vi "com_test.vi"() -> ()   [LabVIEW 2012]
uses:
  <vilib>/Analysis/2dsp.llb/1D Auto Correlation (CDB).vi
  <vilib>/Analysis/2dsp.llb/1D Cross Correlation (CDB).vi
  <vilib>/Analysis/NI_AALPro.lvlib
panel:
  out "Transmitted signal":dbl[](graph)
  out "Transmitted symbols autocorrelation":dbl[](graph)
  out "Transmitted and received symbols Xcorrelation":dbl[](graph)
  out "error out":errorcluster
  in  "RX Parameters":T1={"RX Oversample Factor"=4, "RX Sample Rate"=4000000.0, "Synchronization Options"={"Synchronization Method"=enum."Timing Estimation", "Symbol Timing Recovery Method "=enum."Maximum Energy", "Fixed Offset"=0.0, "Frame Detection Method"=enum."", "Correct Frequency Offset"=FALSE}, "Channel Estimation/Equalization Parameters"={"Equalization Method"=enum."", "Channel Estimate Length"=0.0, "Equalizer Length"=0.0, "Equalizer Delay"=0.0}}
  in  "TX/RX Shared Parameters":T2={"Modulation Type"=enum."FSK", "Packet Length"=128, "# of Iterations"=0.0, "Pulse Shaping Parameters"={"Pulse Shaping Filter"=enum."Gaussian", "Filter Length (symbols)"=8, "Filter Parameter"=0.5, "modulation type"=enum."FSK"}, "Header/Tail Control Information"={"Training Sequence Type"=enum."", "Zero Pad Length"=0.0}}
  out "recovered bits":i32[](array[numeric])
  out "output bit stream":u8[](array[numeric])
  in  "Symbol Energy":dbl=1.0 format="%#_4p"
  in  "Source Type":enum16{"Random Bits", "File"}(ring)
  out "BER":dbl
  in  "Sync Words":i32[](array[numeric])=[1, 1, 1, 0, 0, 1, 0]
  in  "Preamble Length (bits)":u32=20
  in  "TX Parameters":T3={"TX Oversample Factor"=4, "TX Sample Rate"=4000000.0}
  in  "error in (no error)":errorcluster
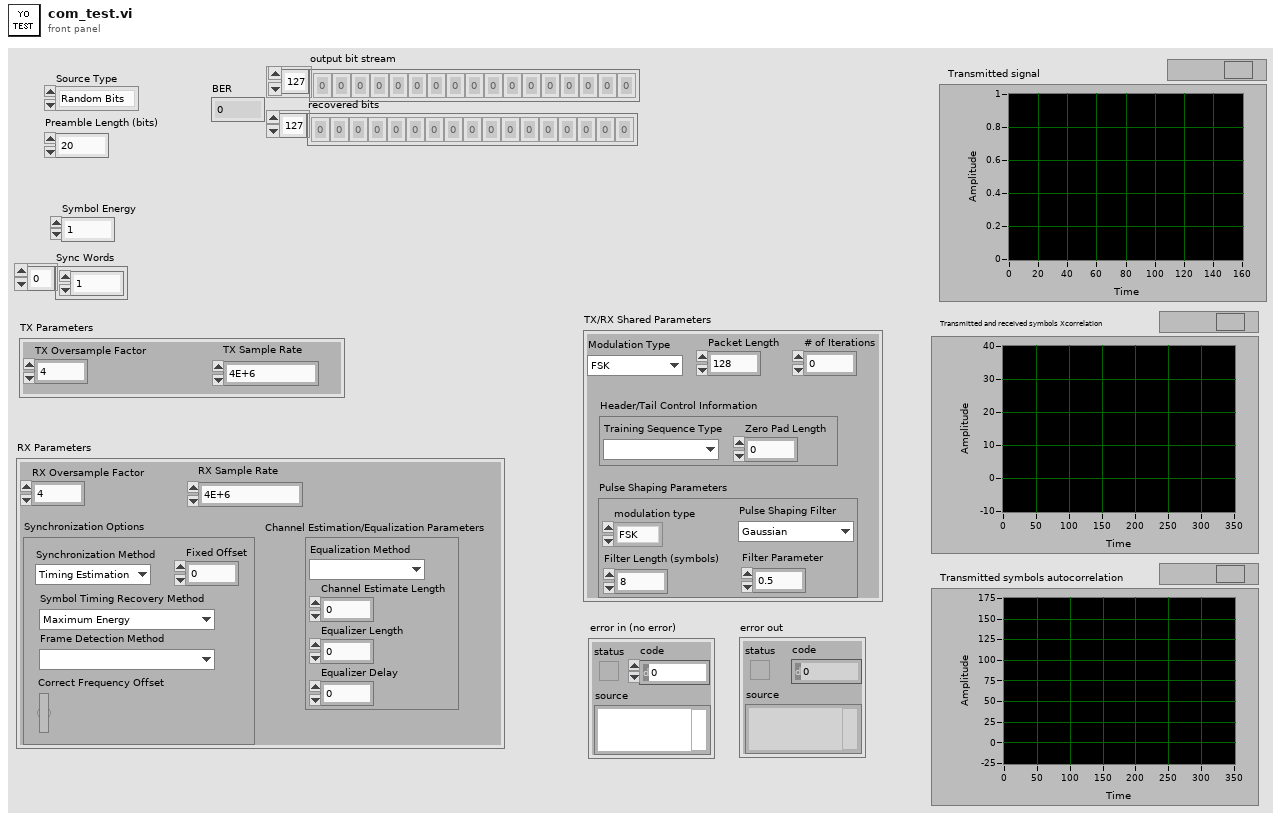
[diagram p1: front panel]
types:
  T1 = cluster{"RX Oversample Factor":i32, "RX Sample Rate":dbl, "Synchronization Options":cluster{"Synchronization Method":enum16{"Fixed Offset", "Timing Estimation", "Joint Timing and Channel Estimation"}, "Symbol Timing Recovery Method ":enum16{"MT Allign To Ideal Symbols", "Maximum Energy", "Early-Late Gate", "Gardner", "Fixed Offset"}, "Fixed Offset":dbl, "Frame Detection Method":enum16{""}, "Correct Frequency Offset":bool}, "Channel Estimation/Equalization Parameters":cluster{"Equalization Method":enum16{""}, "Channel Estimate Length":dbl, "Equalizer Length":dbl, "Equalizer Delay":dbl}}
  T2 = cluster{"Modulation Type":enum16{"OOK", "FSK"}, "Packet Length":i32, "# of Iterations":dbl, "Pulse Shaping Parameters":cluster{"Pulse Shaping Filter":enum16{"none", "Raised Cosine", "Root Raised Cos", "Gaussian"}, "Filter Length (symbols)":i32, "Filter Parameter":dbl, "modulation type":enum16{"FSK", "PSK", "QAM", "MSK", "PAM", "ASK", "CPM"}}, "Header/Tail Control Information":cluster{"Training Sequence Type":enum16{""}, "Zero Pad Length":dbl}}
  T3 = cluster{"TX Oversample Factor":i32, "TX Sample Rate":dbl}
  T4 = cluster{"TX Parameters":cluster{"TX Oversample Factor":i32, "TX Sample Rate":dbl}, "TX/RX Shared Parameters":cluster{"Modulation Type":enum16{"OOK", "FSK"}, "Packet Length":i32, "# of Iterations":dbl, "Pulse Shaping Parameters":cluster{"Pulse Shaping Filter":enum16{"none", "Raised Cosine", "Root Raised Cos", "Gaussian"}, "Filter Length (symbols)":i32, "Filter Parameter":dbl, "modulation type":enum16{"FSK", "PSK", "QAM", "MSK", "PAM", "ASK", "CPM"}}, "Header/Tail Control Information":cluster{"Training Sequence Type":enum16{""}, "Zero Pad Length":dbl}}}
  T5 = cluster{"RX Parameters":cluster{"RX Oversample Factor":i32, "RX Sample Rate":dbl, "Synchronization Options":cluster{"Synchronization Method":enum16{"Fixed Offset", "Timing Estimation", "Joint Timing and Channel Estimation"}, "Symbol Timing Recovery Method ":enum16{"MT Allign To Ideal Symbols", "Maximum Energy", "Early-Late Gate", "Gardner", "Fixed Offset"}, "Fixed Offset":dbl, "Frame Detection Method":enum16{""}, "Correct Frequency Offset":bool}, "Channel Estimation/Equalization Parameters":cluster{"Equalization Method":enum16{""}, "Channel Estimate Length":dbl, "Equalizer Length":dbl, "Equalizer Delay":dbl}}, "TX/RX Shared Parameters":cluster{"Modulation Type":enum16{"OOK", "FSK"}, "Packet Length":i32, "# of Iterations":dbl, "Pulse Shaping Parameters":cluster{"Pulse Shaping Filter":enum16{"none", "Raised Cosine", "Root Raised Cos", "Gaussian"}, "Filter Length (symbols)":i32, "Filter Parameter":dbl, "modulation type":enum16{"FSK", "PSK", "QAM", "MSK", "PAM", "ASK", "CPM"}}, "Header/Tail Control Information":cluster{"Training Sequence Type":enum16{""}, "Zero Pad Length":dbl}}}
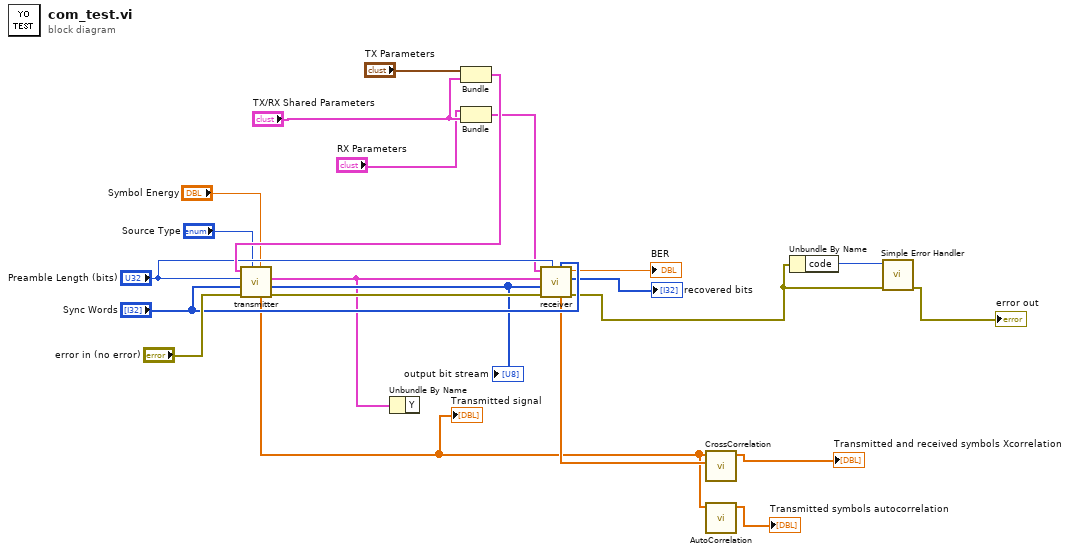
[diagram p0: block diagram]
diagram:
  n1 = Bundle("TX Parameters"="TX Parameters", "TX/RX Shared Parameters"="TX/RX Shared Parameters") -> (w19:T4)  [unwired: 1 in]
  n2 = call "transmitter.vi"("Symbol Energy"="Symbol Energy", "Source Type"="Source Type", "error in (no error)"="error in (no error)", "Sync Words"="Sync Words", "Preamble Length (bits)"="Preamble Length (bits)", "Modulation Parameters In"=w19) -> ("error out"=w22:errorcluster, "output bit stream"=w10:u8[], "output MT waveform"=w5:cluster{"t0":dbl, "dt":dbl, "Y":cdb[]}, "Output Symbols"=w4:cdb[])  [unwired: 1 in, 1 out]
  "output bit stream" <- w10
  "Transmitted signal" <- w4
  n3 = Unbundle By Name(w5) -> ()  [unwired: 1 out]
  n4 = Bundle("RX Parameters"="RX Parameters", "TX/RX Shared Parameters"="TX/RX Shared Parameters") -> (w12:T5)  [unwired: 1 in]
  n5 = call "receiver.vi"("Sync Words"="Sync Words", "preamble length"="Preamble Length (bits)", "error in (no error)"=w22, "Key Bit Sequence"=w10, "input complex waveform"=w5, "Modulation Parameters In"=w12) -> ("error out"=w2:errorcluster, "recovered bits"=→"recovered bits":i32[], "BER"=→"BER":dbl, "Recovered Symbols"=w8:cdb[])  [unwired: 2 in]
  n6 = call-poly <vilib>:"CrossCorrelation.vi"("Y"=w8, "X"=w4) -> ("Rxy"=→"Transmitted and received symbols Xcorrelation":cdb[])  [unwired: 8 in, 1 out]
  n7 = call-poly <vilib>:"AutoCorrelation.vi"("X"=w4) -> ("Rxx"=→"Transmitted symbols autocorrelation":cdb[])  [unwired: 9 in, 1 out]
  n8 = Unbundle By Name(w2) -> ("code"=w3:i32)
  n9 = call <vilib>:"Simple Error Handler.vi"("error code (no error:0)"=w3, "error in (no error)"=w2) -> ("error out"=→"error out":errorcluster)  [unwired: 3 in, 4 out]
